vi "compy.vi"(8 "error in":errorcluster, 10 "Commands Queue":refnum<queue>, 11 "User Event Ref IN":refnum<user-event>) -> (0 "error out":errorcluster)   [LabVIEW 2022 SP3]
panel:
  in  "Py Script Connect":bool
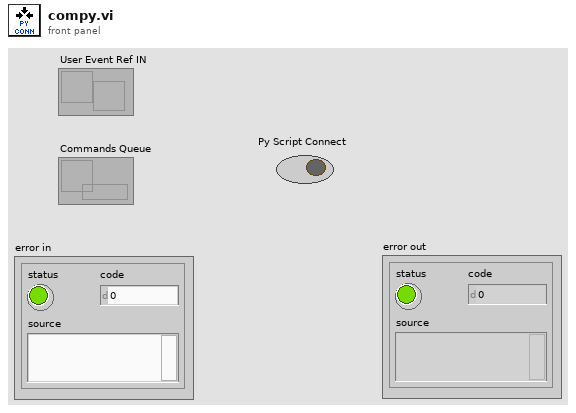
[diagram p1: front panel]
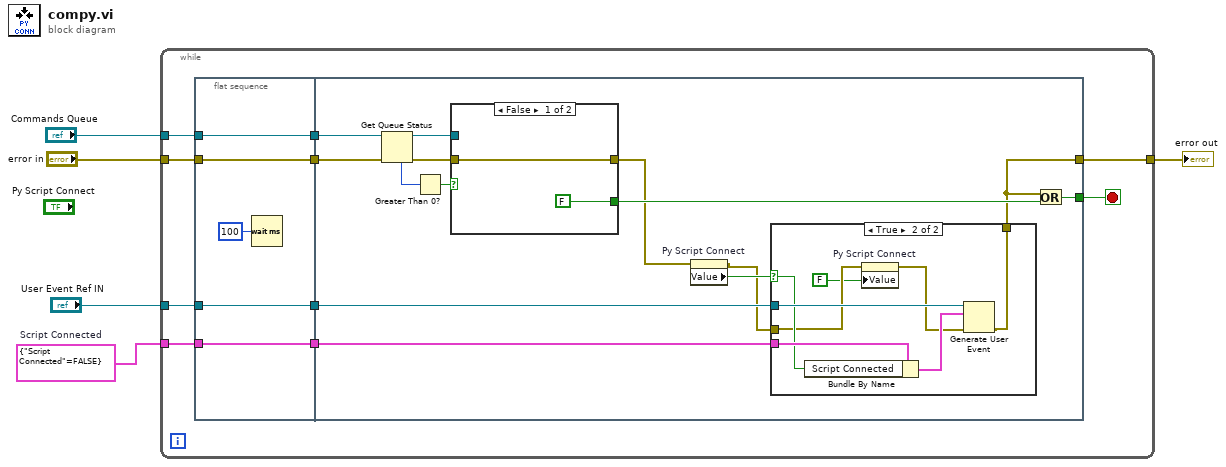
[diagram p0: block diagram]
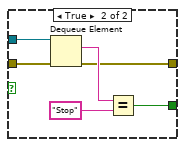
[diagram p3: hidden frame]
diagram:
  w1 = cluster{"Script Connected":bool} {"Script Connected"=FALSE}  # Script Connected
  n1 = while {
    tunnel: "Commands Queue" -> [w15]
    tunnel: "error in" -> [w13]
    tunnel: [w10] -> w3
    tunnel: "User Event Ref IN" -> [w12]
    tunnel: w1 -> [w11]
    stop <- w14 stop-if-true
    n2 = flat-sequence {
      tunnel: w11 -> [w17]
      tunnel: w12 -> [w18]
      tunnel: w13 -> [w19]
      tunnel: w15 -> [w20]
      tunnel: [w20] -> w9
      tunnel: [w19] -> w8
      tunnel: [w18] -> w7
      tunnel: [w17] -> w6
      tunnel: [w28] -> w14
      tunnel: [w21] -> w10
      tunnel: w9 -> [w34]
      tunnel: w8 -> [w27]
      tunnel: w7 -> [w24]
      tunnel: w6 -> [w22]
      frame #0 {
        n3 = Wait (ms)(milliseconds to wait=u32 100) -> ()  [unwired: 1 out]
      }
      frame #1 {
        n4 = Get Queue Status(queue=w34, error in (no error)=w27) -> (queue out=w30:refnum<queue>, error out=w31:errorcluster, # elements in queue=w33:i32)  [unwired: 1 in, 5 out]
        n5 = Greater Than 0?(x=w33) -> (x > 0?=w32:bool)
        n6 = case shown="False" w32 {
          tunnel: w31 -> [w44 w51]
          tunnel: w30 -> [_ w50]
          tunnel: [w44 w48] -> w26
          tunnel: [FALSE w46] -> w29
          frame False {
          }
          frame True {
            n7 = Dequeue Element(queue=w50, error in (no error)=w51) -> (element=w49:string, error out=w48:errorcluster)  [unwired: 1 in, 2 out]
            n8 = Equal?(x=w49, y="Stop") -> (x = y?=w46:bool)
          }
        }
        n9 = property on="Py Script Connect" class="Bool (strict)"(error in=w26) -> (error out=w23:errorcluster, "Value"=w25:bool)  [unwired: 1 in, 1 out]
        n10 = case shown="True" w25 {
          selector: w25 -> [_ w41]
          tunnel: w24 -> [_ w43]
          tunnel: w23 -> [w35 w38]
          tunnel: w22 -> [_ w42]
          tunnel: [w35 w39] -> w21
          frame False {
          }
          frame True {
            n11 = Bundle By Name(cluster=w42, "Script Connected"=w41) -> (w40:cluster{"Script Connected":bool})
            n12 = property on="Py Script Connect" class="Bool (strict)"(error in=w38, "Value"=FALSE ("Py Script Connect")) -> (error out=w37:errorcluster)  [unwired: 1 in, 1 out]
            n13 = Generate User Event(user event=w43, event data cluster=w40, error in=w37) -> (error out=w39:errorcluster)  [unwired: 1 in, 1 out]
          }
        }
        n14 = Or(x=w21, y=w29) -> (x .or. y?=w28:bool)
      }
    }
  }
  "error out" <- w3
